vi "Create File if not present.vi"(0 "Error Logger Path":path, 11 "error in (no error)":errorcluster) -> (4 "Duplicate Path":path, 15 "error out":errorcluster)   [LabVIEW 2021, in "Path Functions.lvlib"]
uses:
  Path Functions.lvlib
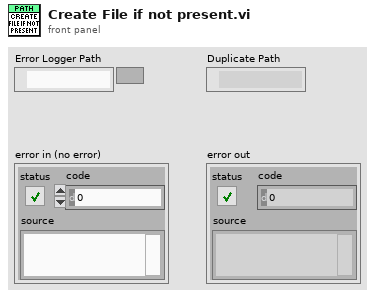
[diagram p1: front panel]
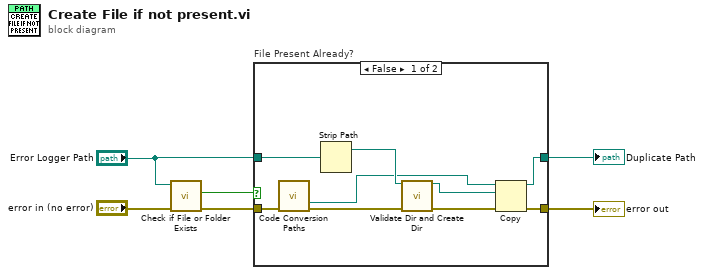
[diagram p0: block diagram]
diagram:
  n1 = call <vilib>:"Check if File or Folder Exists.vi"("error in (no error)"="error in (no error)", "path"="Error Logger Path") -> ("error out"=w2:errorcluster, "file or folder exists?"=w3:bool)  [unwired: 7 in, 1 out]
  n2 = case "File Present Already?" shown="False" w3 {
    tunnel: w2 -> [w14 w17]
    tunnel: "Error Logger Path" -> [w15 w16]
    tunnel: [w13 w17] -> w6
    tunnel: [w7 w16] -> w1
    frame False {
      n3 = call "Code Conversion Paths.vi"("error in (no error)"=w14) -> ("Error Log Path"=w10:path, "error out"=w8:errorcluster)  [unwired: 6 in, 7 out]
      n4 = Strip Path(path=w15) -> (stripped path=w12:path)  [unwired: 1 out]
      n5 = call "Validate Dir and Create Dir.vi"("Directory"=w12, "error in (no error)"=w8) -> ("Dup Directory"=w11:path, "error out"=w9:errorcluster)  [unwired: 12 in]
      n6 = Copy(8:w9, 10:w11, 11:w10) -> (0:w13:errorcluster, 3:w7:path)  [unwired: 2 in, 1 out]
    }
    frame True {
    }
  }
  "error out" <- w6
  "Duplicate Path" <- w1
